vi "szukanie głowy.vi"(11 "Array in":dbl[][](array[numeric])) -> (2 "wiersz":i32, 3 "kolumna":i32)   [LabVIEW 2020]
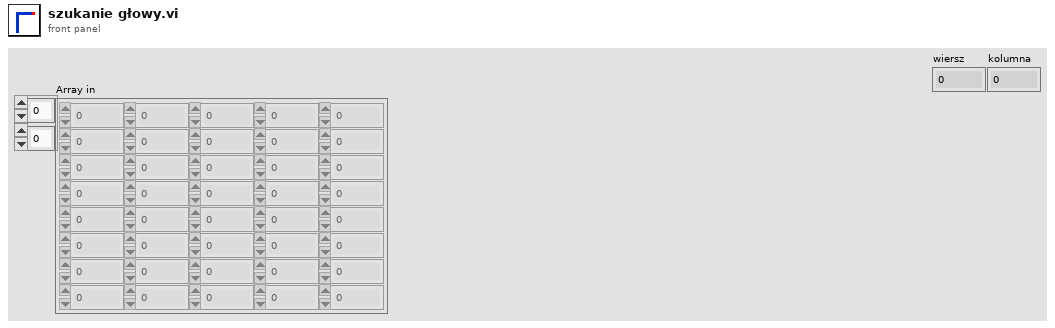
[diagram p1: front panel]
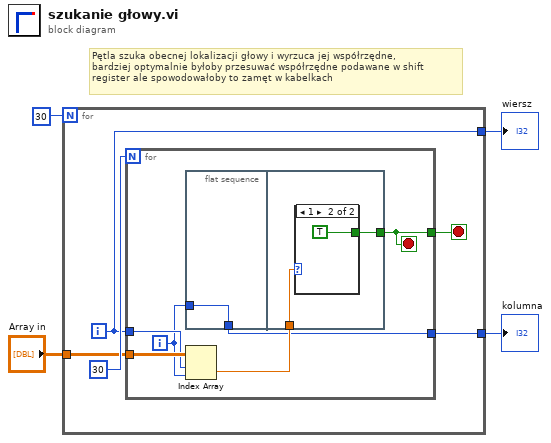
[diagram p0: block diagram]
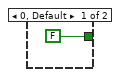
[diagram p2: hidden frame]
diagram:
  # "Pętla szuka obecnej lokalizacji głowy i wyrzuca jej współrzędne, \nbardziej optymalnie byłoby przesuwać współrzędne podawane w shift \nregister ale spowodowałoby to zamęt w kabelkach"
  n1 = for {
    N: 30 -> [_]
    tunnel: "Array in" -> [w8]
    tunnel: [w7] -> w2
    tunnel: [w6] -> w1
    i -> [w6]
    stop <- w5 stop-if-true
    n2 = for {
      N: 30 -> [_]
      tunnel: w8 -> [w15]
      tunnel: w6 -> [w14]
      tunnel: [w11] -> w7
      tunnel: [w10] -> w5
      i -> [w12]
      stop <- w10 stop-if-true
      n3 = flat-sequence {
        tunnel: w12 -> [w16]
        tunnel: [w16] -> w11
        tunnel: w13 -> [w18]
        tunnel: [w17] -> w10
        frame #0 {
        }
        frame #1 {
          n4 = case shown="1" w18 {
            tunnel: [FALSE TRUE] -> w17
            frame 0, Default {
            }
            frame 1 {
            }
          }
        }
      }
      n5 = Index Array(array=w15, index (row)=w14, index (col)=w12) -> (element=w13:dbl)
    }
  }
  "wiersz" <- w1
  "kolumna" <- w2
